vi "Get Build Spec Information.vi"() -> ()   [LabVIEW 2013]
panel:
  out "Array":string[](array[string])
  out "Setup Exe Path":path
  out "Array 2":variant[](array[variant])
  out "Tag:Get Names":string[](array[string])
  out "error out":errorcluster
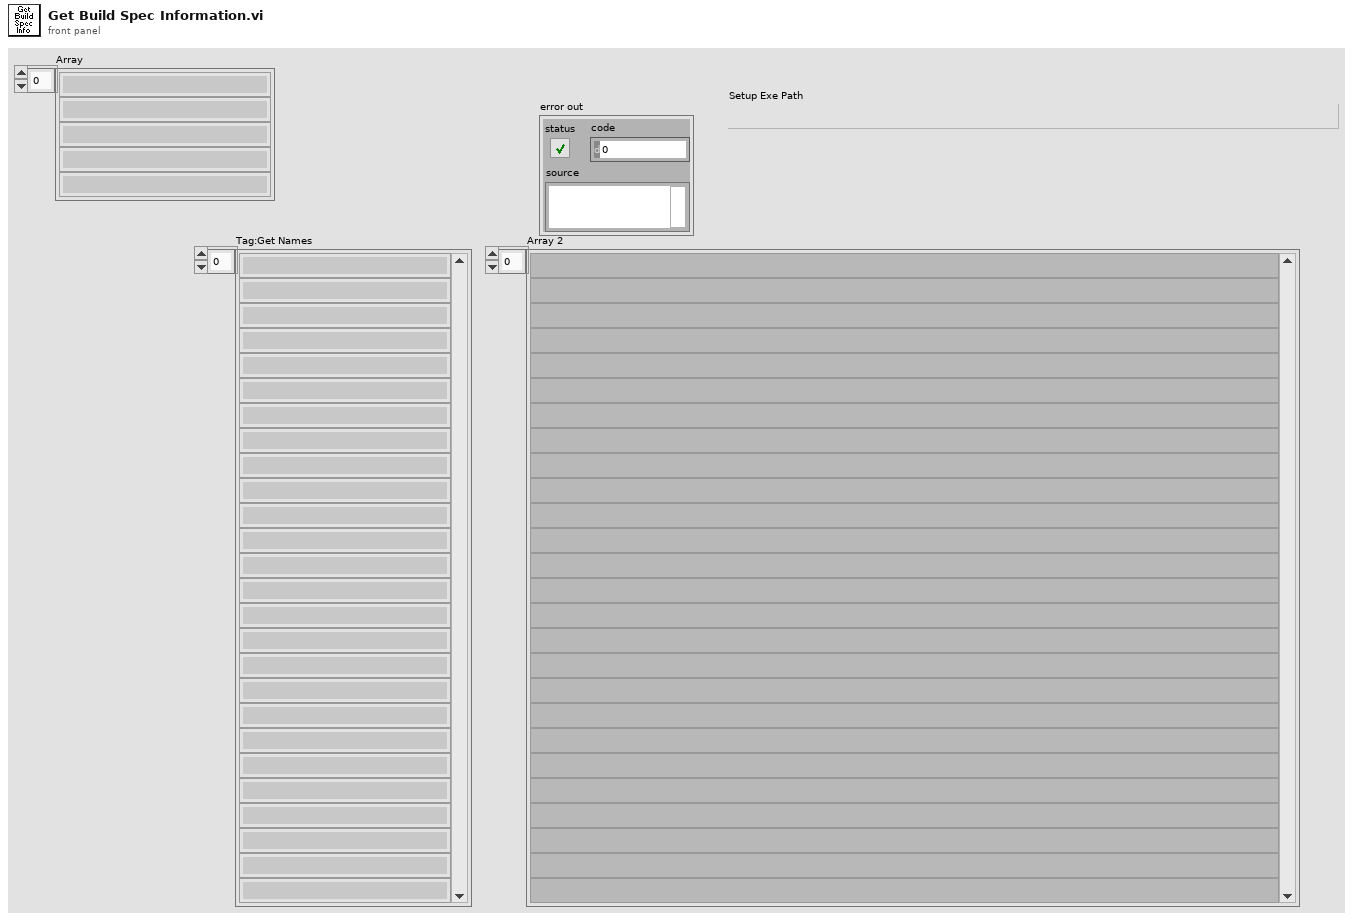
[diagram p1: front panel]
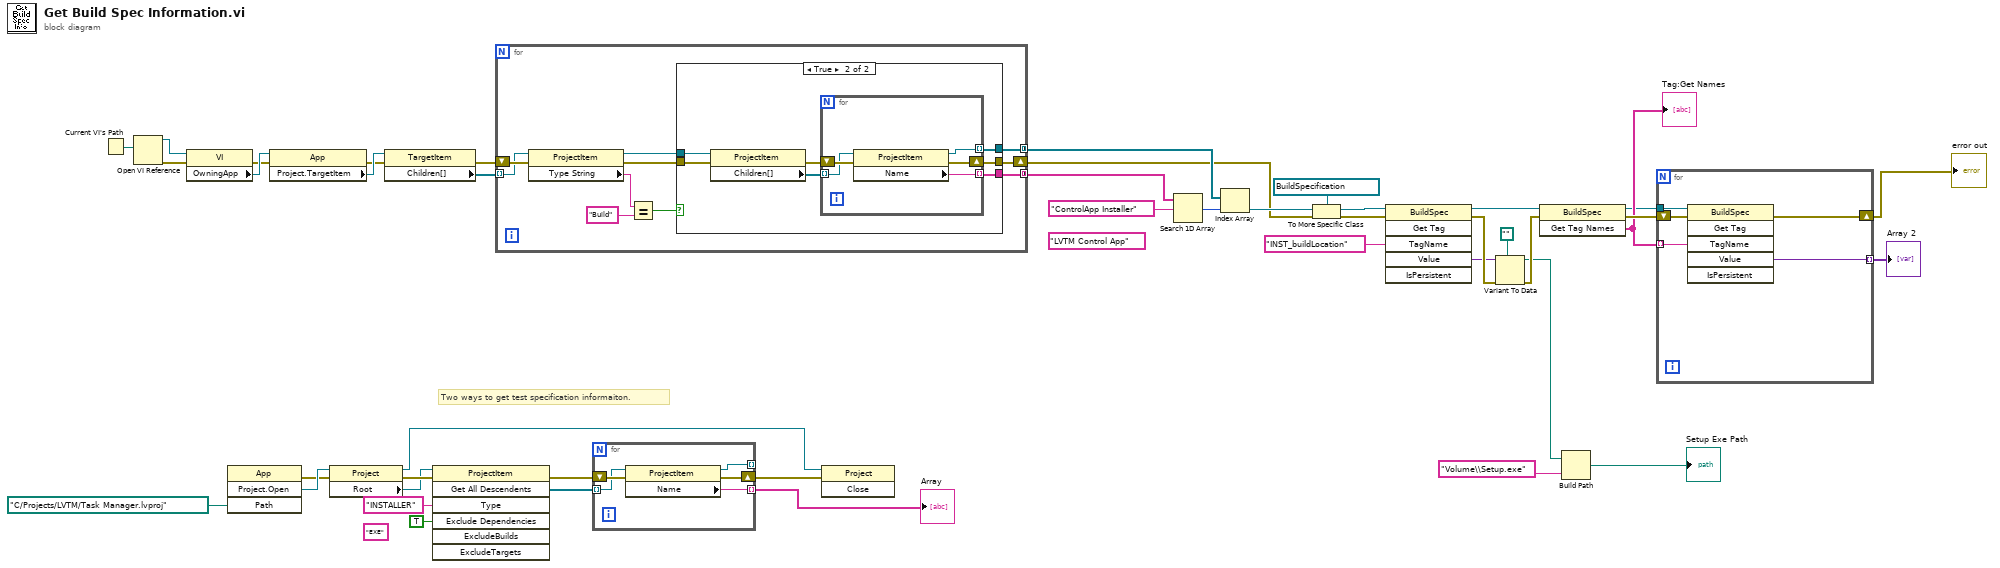
[diagram p0: block diagram]
diagram:
  (unwired) "EXE" ("Type")
  (unwired) "LVTM Control App" ("y")
  # "Two ways to get test specification informaiton."
  n1 = Current VI's Path() -> (path=w44:path)
  n2 = Open VI Reference(vi path=w44) -> (vi reference=w43:refnum<vi>, error out=w42:errorcluster)  [unwired: 5 in]
  n3 = property class="VI"(reference=w43, error in=w42) -> (error out=w40:errorcluster, "OwningApp"=w41:refnum<vi>)  [unwired: 1 out]
  n4 = invoke class="App" method="Project.Open"("Path"=path "C:/Projects/LVTM/Task Manager.lvproj") -> (error out=w10:errorcluster, "Project:Open"=w11:refnum<vi>)  [unwired: 3 in, 2 out]
  n5 = property class="App"(reference=w41, error in=w40) -> (error out=w38:errorcluster, "Project.TargetItem"=w39:refnum<vi>)  [unwired: 1 out]
  n6 = property class="Project"(reference=w11, error in=w10) -> (reference out=w2:refnum<vi>, error out=w9:errorcluster, "Root"=w8:refnum<vi>)
  n7 = property class="TargetItem"(reference=w39, error in=w38) -> (error out=w36:errorcluster, "Children[]"=w37:refnum<vi>[])  [unwired: 1 out]
  n8 = invoke class="ProjectItem" method="Get All Descendents"(reference=w8, error in=w9, "Type"="INSTALLER", "Exclude Dependencies"=TRUE ("ExcludeDependencies")) -> (error out=w4:errorcluster, "All Descendents"=w5:refnum<vi>[])  [unwired: 3 in, 5 out]
  n9 = for {
    tunnel: w37 -> [w53] mode=indexing
    shift-right: [w48] -> w29
    shift-left: w36 -> [w54]
    tunnel: [w46] -> w35 mode=concatenating
    tunnel: [w45] -> w33 mode=concatenating
    n10 = property class="ProjectItem"(reference=w53, error in=w54) -> (reference out=w50:refnum<vi>, error out=w49:errorcluster, "Type String"=w52:string)
    n11 = Equal?(x=w52, y="Build") -> (x = y?=w47:bool)
    n12 = case shown="True" w47 {
      tunnel: w50 -> [_ w60]
      tunnel: w49 -> [w55 w59]
      tunnel: [w55 w58] -> w48
      tunnel: [_ w57] -> w46
      tunnel: [_ w56] -> w45
      frame False {
      }
      frame True {
        n13 = property class="ProjectItem"(reference=w60, error in=w59) -> (error out=w61:errorcluster, "Children[]"=w62:refnum<vi>[])  [unwired: 1 out]
        n14 = for {
          tunnel: w62 -> [w66] mode=indexing
          shift-right: [w65] -> w58
          shift-left: w61 -> [w67]
          tunnel: [w64] -> w57 mode=indexing
          tunnel: [w63] -> w56 mode=indexing
          n15 = property class="ProjectItem"(reference=w66, error in=w67) -> (reference out=w63:refnum<vi>, error out=w65:errorcluster, "Name"=w64:string)
        }
      }
    }
  }
  n16 = for {
    tunnel: w5 -> [w71] mode=indexing
    shift-right: [w70] -> w1
    shift-left: w4 -> [w72]
    tunnel: [w69] -> w3 mode=indexing
    tunnel: [w68] -> _ mode=indexing
    n17 = property class="ProjectItem"(reference=w71, error in=w72) -> (reference out=w68:refnum<vi>, error out=w70:errorcluster, "Name"=w69:string)
  }
  "Array" <- w3
  n18 = invoke class="Project" method="Close"(reference=w2, error in=w1) -> ()  [unwired: 1 in, 3 out]
  n19 = Search 1D Array(1D array=w35, element="ControlApp Installer" ("y")) -> (index of element=w32:i32)  [unwired: 1 in]
  n20 = Index Array(array=w33, index=w32) -> (element=w31:refnum<vi>)
  n21 = To More Specific Class(target class=refnum<vi> refnum ("element"), reference=w31, error in=w29) -> (specific class reference=w20:refnum<vi>, error out=w18:errorcluster)
  n22 = invoke class="BuildSpec" method="Get Tag"(reference=w20, error in=w18, "TagName"="INST_buildLocation" ("y")) -> (reference out=w19:refnum<vi>, error out=w23:errorcluster, "Value"=w22:variant)  [unwired: 3 in, 3 out]
  n23 = Variant To Data(error in=w23, type=path "", Variant=w22) -> (data=w16:path, error out=w17:errorcluster)
  n24 = invoke class="BuildSpec" method="Get Tag Names"(reference=w19, error in=w17) -> (reference out=w24:refnum<vi>, error out=w28:errorcluster, "Get Tag Names"=w26:string[])  [unwired: 1 in]
  "Tag:Get Names" <- w26
  n25 = Build Path(base path=w16, name or relative path="Volume\\Setup.exe" ("string")) -> (appended path=→"Setup Exe Path":path)
  n26 = for {
    tunnel: w24 -> [w77]
    tunnel: w26 -> [w75] mode=indexing
    tunnel: [w74] -> w27 mode=indexing
    shift-right: [w73] -> w13
    shift-left: w28 -> [w76]
    n27 = invoke class="BuildSpec" method="Get Tag"(reference=w77, error in=w76, "TagName"=w75) -> (error out=w73:errorcluster, "Value"=w74:variant)  [unwired: 3 in, 4 out]
  }
  "error out" <- w13
  "Array 2" <- w27
